vi "Load tear.vi"() -> (1 "Load Cell":dbl)   [LabVIEW 2020]
uses:
  Galobal variable_TI.vi
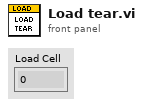
[diagram p1: front panel]
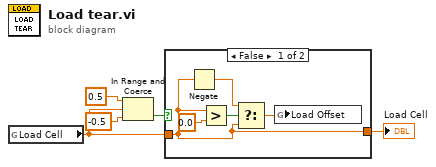
[diagram p0: block diagram]
diagram:
  n1 = global read "Galobal variable_TI.vi" "Load Cell"() -> (w5:dbl)
  n2 = In Range and Coerce(upper limit=0.5, x=w5, lower limit=-0.5) -> (In Range?=w2:bool)  [unwired: 1 out]
  n3 = case shown="False" w2 {
    tunnel: w5 -> [w6 w11]
    tunnel: [w6 w11] -> w1
    frame False {
      n4 = Negate(x=w6) -> (-x=w8:dbl)
      n5 = Greater?(x=w6, y=0.0) -> (0:w9:bool)
      n6 = Select(t=w8, s=w9, f=w6) -> (s? t:f=w7:dbl)
      n7 = global write "Galobal variable_TI.vi" "Load Offset"(w7) -> ()
    }
    frame True {
    }
  }
  "Load Cell" <- w1
